vi "Serialize - JSON.vi"(8 "error in":errorcluster, 11 "Heater Data in":refnum<class "Heater Data.lvclass">) -> (0 "error out":errorcluster, 2 "Serialized JSON":string, 3 "Heater Data out":refnum<class "Heater Data.lvclass">)   [LabVIEW 2017, in "Controller.lvlib" / "Heater Data.lvclass"]
uses:
  Heater Data.lvclass
  C:/Program Files (x86)/National Instruments/LabVIEW 2017/vi.lib/MSR Consulting, LLC/General Reuse/Data/Data.lvclass
  <vilib>/MSR Consulting, LLC/General Reuse/Data/Data.lvclass/Data.ctl
  Heater Data.lvclass/Heater Data.ctl
  <vilib>/MSR Consulting, LLC/General Reuse/Data/Read Data ID.vi
  <vilib>/MSR Consulting, LLC/General Reuse/Data/Data.lvclass
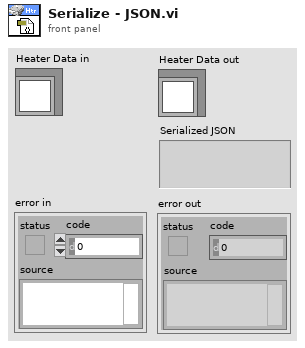
[diagram p1: front panel]
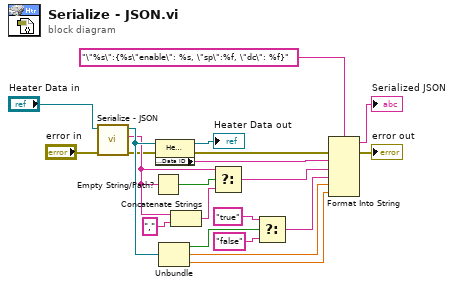
[diagram p0: block diagram]
diagram:
  n1 = call-parent "Serialize - JSON.vi"("error in"="error in", "Data in"="Heater Data in") -> ("error out"=w3:errorcluster, "Serialized JSON"=w11:string, "Data out"=w15:refnum<class "Heater Data.lvclass">)  [unwired: 7 in]
  n2 = Empty String/Path?(string/path=w11) -> (empty?=w12:bool)
  n3 = property class="Heater Data"(reference=w15, error in=w3) -> (reference out=→"Heater Data out":refnum<class "Heater Data.lvclass">, error out=w2:errorcluster, "Accessors:Data ID"=w10:string)
  n4 = Unbundle(w15) -> (w17:bool, w7:dbl, w6:dbl)
  n5 = Concatenate Strings(w11, "," ("string")) -> (w13:string)
  n6 = Select(t=w11, s=w12, f=w13) -> (s? t:f=w9:string)
  n7 = Select(t="true", s=w17, f="false") -> (s? t:f=w8:string)
  n8 = Format Into String(format string="\"%s\":{%s\"enable\": %s, \"sp\":%f, \"dc\": %f}", error in=w2, w10, w9, w8, w7, w6) -> (resulting string=→"Serialized JSON":string, error out=→"error out":errorcluster)  [unwired: 1 in]
